vi "MarbleDispenserMk3.vi"   [LabVIEW 2016]
uses:
  <vilib>/NXT/Block Support/NXT_InputPort.ctl
  <vilib>/NXT/Block Support/NXT_OutputPort.ctl
  <vilib>/NXT/Dual Mode Library/Sensors/Touch_Released.vi
  <vilib>/NXT/NXTIO Xnodes/NXTIONodeSubVIs/NXTStopMotors.vi
  <vilib>/NXT/NXTIO Xnodes/NXTIONodeSubVIs/NXTMoveMotors.vi
  <vilib>/NXT/NXTIO Xnodes/NXTIONodeSubVIs/NXTMotorRunDistance.vi
  <vilib>/NXT/Dual Mode Library/Waits/Wait_Num.vi
  <vilib>/NXT/Subs/LVHSConnector.ctl
  <vilib>/NXT/NXTIO Xnodes/AddressXNode/NXTIOAddress.xnode
  <vilib>/NXT/NXTIO Xnodes/NXTIOXNode/NXTIO.xnode
  <vilib>/NXT/LegoClasses/BrickReference/BrickReference.lvclass
types:
  T1 = typedef "NXT_InputPort.ctl" = u32
  T2 = typedef "NXT_OutputPort.ctl" = u8
  T3 = typedef "LVHSConnector.ctl" = refnum<class "BrickReference.lvclass">
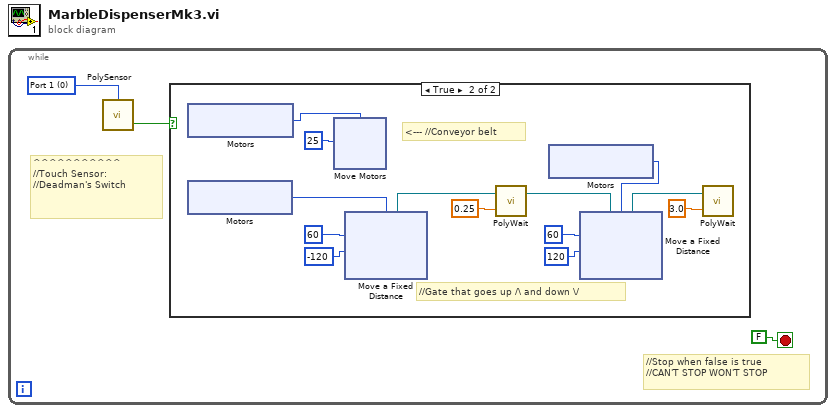
[diagram p0: block diagram]
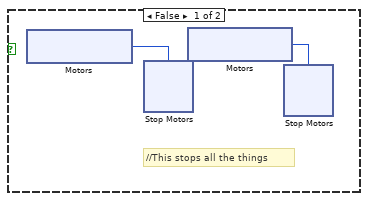
[diagram p2: hidden frame]
diagram:
  n1 = while {
    stop <- FALSE stop-if-true
    w3 = T1 0 items=["Port 1", "Port 2", "Port 3", "Port 4"] ("Port (Port 1)")
    # "//Stop when false is true\n//CAN'T STOP WON'T STOP"
    # "^^^^^^^^^^^\n//Touch Sensor:\n//Deadman's Switch"
    n2 = call-poly <vilib>:"PolySensor.vi"("Port (Port 1)"=w3) -> ("Yes / No"=w1:bool)  [unwired: 2 in, 1 out]
    n3 = case shown="True" w1 {
      frame False {
        # "//This stops all the things"
        n4 = xnode "Motors"() -> ("Motor"=w5:T2)
        n5 = xnode "Stop Motors"("Motors"=w5) -> ()  [unwired: 1 in, 1 out]
        n6 = xnode "Motors"() -> ("Motor"=w4:T2)
        n7 = xnode "Stop Motors"("Motors"=w4) -> ()  [unwired: 1 in, 1 out]
      }
      frame True {
        # "//Gate that goes up /\\ and down \\/"
        # "<--- //Conveyor belt"
        n8 = xnode "Motors"() -> ("Motor"=w30:T2)
        n9 = xnode "Motors"() -> ("Motor"=w24:T2)
        n10 = xnode "Move Motors"("Power/Speed 1"=25, "Motors"=w30) -> ()  [unwired: 1 in, 1 out]
        n11 = xnode "Move a Fixed Distance"("Speed 1"=-120, "Distance 1"=60, "Motors"=w24) -> ("NXT/EV3"=w27:T3)  [unwired: 1 in]
        n12 = call-poly <vilib>:"PolyWait.vi"("Time (1 sec)"=0.25, "NXT/EV3"=w27) -> ("NXT/EV3"=w19:T3)  [unwired: 2 in]
        n13 = xnode "Motors"() -> ("Motor"=w18:T2)
        n14 = xnode "Move a Fixed Distance"("Speed 1"=120, "Distance 1"=60, "Motors"=w18, "NXT/EV3"=w19) -> ("NXT/EV3"=w22:T3)
        n15 = call-poly <vilib>:"PolyWait.vi"("Time (1 sec)"=3.0, "NXT/EV3"=w22) -> ()  [unwired: 2 in, 1 out]
      }
    }
  }
